vi "IsAttrMap.vi"(11 "Variant":variant) -> (2 "KeyMap":T2, 3 "True":bool, 5 "AttrMap":T1)   [LabVIEW 2019, in "lv-apt-json-file.lvlib"]
uses:
  lv-apt-json-file.lvlib
  Typedef/Def-AttrMap -- NameMap.ctl
  Typedef/Def-AttrMap.ctl
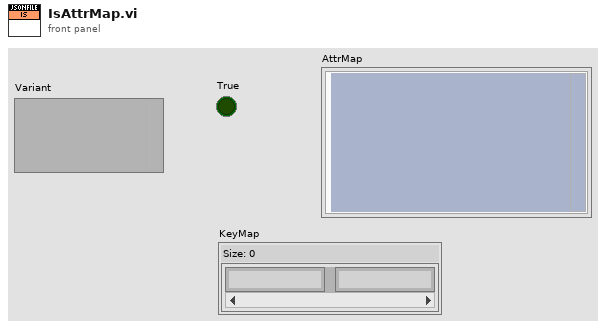
[diagram p1: front panel]
types:
  T1 = typedef "lv-apt-json-file.lvlib/Def-AttrMap.ctl" = cluster{"Map":variant}
  T2 = typedef "lv-apt-json-file.lvlib/Def-AttrMap -- NameMap.ctl" = map{string, string}
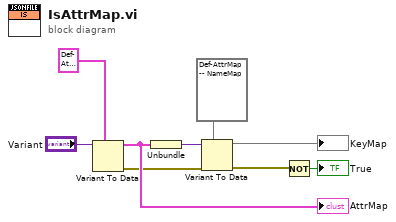
[diagram p0: block diagram]
diagram:
  n1 = Variant To Data(type=T1 {"Map"=variant} ("Enum"), Variant="Variant") -> (data=w6:T1, error out=w2:errorcluster)  [unwired: 1 in]
  "AttrMap" <- w6
  n2 = Unbundle(w6) -> ("Map"=w5:variant)
  n3 = Variant To Data(error in=w2, type=T2 {} ("AttrMap"), Variant=w5) -> (data=→"KeyMap":T2, error out=w1:errorcluster)
  n4 = Not(x=w1) -> (.not. x?=→"True":bool)
